vi "Read Test Data.vi"   [LabVIEW 2020, in "eec 6700.lvlib"]
doc: "Reads the test data from the instrument."
uses:
  <instrlib>/eec 6700/eec 6700.lvlib
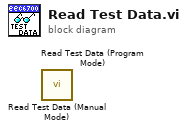
[diagram p0: block diagram]
diagram:
  n1 = call <instrlib>:"Read Test Data (Manual Mode).vi"() -> ()  [unwired: 13 in, 3 out]
  n2 = call <instrlib>:"Read Test Data (Program Mode).vi"() -> ()  [unwired: 13 in, 3 out]
